vi "Set_SglVar_BulkMode_Value.vi"(8 "error in (no error)":errorcluster, 9 "varValue":dbl[](array[numeric]) format="%#_13g", 11 "mupExpr in":refnum<data-value>) -> (0 "error out":errorcluster, 3 "mupExpr out":refnum<data-value>)   [LabVIEW 2015, in "mupExpr.lvclass"]
doc: "Set the bulk mode values of the expression's single variable.\n\nIf the expression contains no variables, the input value is ignored."
uses:
  mupExpr.lvclass
  mupExpr.lvclass/mupExpr.ctl
  mupLib/mupLib.lvlib
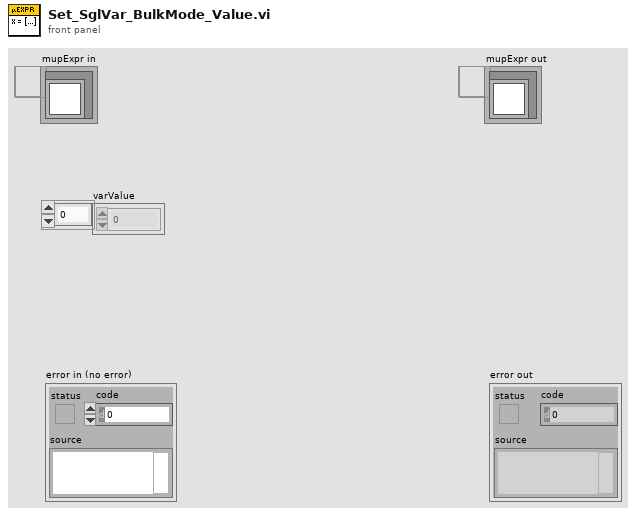
[diagram p1: front panel]
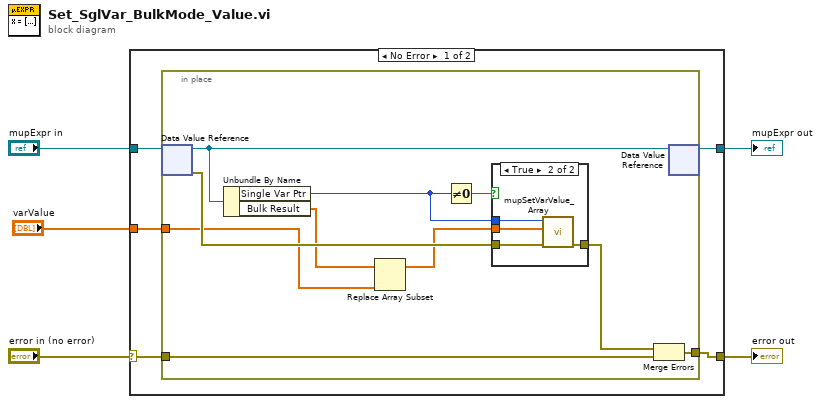
[diagram p0: block diagram]
diagram:
  n1 = case shown="No Error" "error in (no error)" {
    selector: "error in (no error)" -> [w6 w26]
    tunnel: "varValue" -> [w10 _]
    tunnel: "mupExpr in" -> [w9 w27]
    tunnel: [w8 w26] -> w3
    tunnel: [w7 w27] -> w2
    frame No Error {
      n2 = in-place {
        in-place-border: w6 -> [w16]
        in-place-border: w10 -> [w12]
        in-place-border: [w20] -> w8
        n3 = in-place-dvr #1(w9) -> (w19:refnum<class "mupExpr.lvclass">, w15:errorcluster)
        n4 = Unbundle By Name(w19) -> ("Single Var Ptr"=w17:u64, "Bulk Result"=w13:dbl[])
        n5 = Replace Array Subset(array=w13, new element=w12) -> (w11:dbl[])  [unwired: 1 in]
        n6 = Not Equal To 0?(x=w17) -> (x != 0?=w18:bool)
        n7 = case shown="True" w18 {
          tunnel: w17 -> [_ w25]
          tunnel: w11 -> [_ w24]
          tunnel: w15 -> [w21 w23]
          tunnel: [w21 w22] -> w14
          frame False {
          }
          frame True {
            n8 = call "mupSetVarValue_Array.vi"("error in (no error)"=w23, "varValue"=w24, "varPtr in"=w25) -> ("error out"=w22:errorcluster)  [unwired: 7 in, 1 out]
          }
        }
        n9 = Merge Errors(w14, w16) -> (w20:errorcluster)
        n10 = in-place-dvr #1(w19) -> (w7:refnum<data-value>)  [unwired: 1 out]
      }
    }
    frame Error {
    }
  }
  "error out" <- w3
  "mupExpr out" <- w2
